vi "ConfigParseProgram.vi"(8 "error in (no error)":errorcluster, 10 "node result array":refnum<k20>[](array[refnum])) -> (0 "error out":errorcluster, 3 "Program Array":string[][](array[string]))   [LabVIEW 2018, in "Config.lvlib"]
uses:
  Config.lvlib
  <vilib>/xml/NI_XML.lvlib
  <resource>/objmgr/DOMUserDefRef.rc
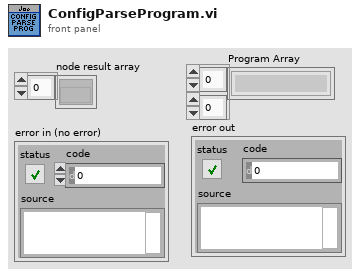
[diagram p1: front panel]
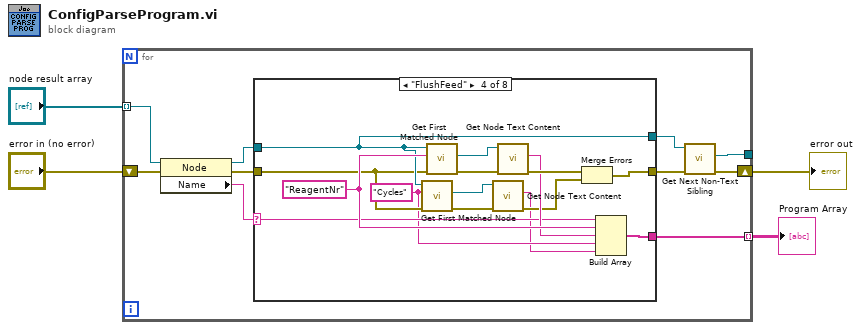
[diagram p0: block diagram]
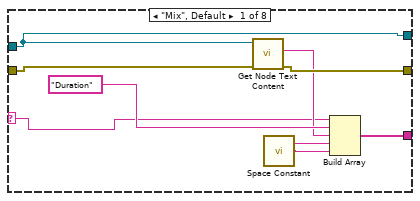
[diagram p2: hidden frame]
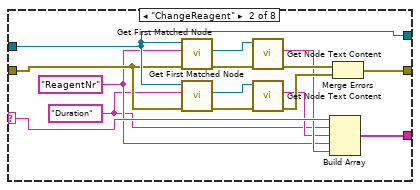
[diagram p3: hidden frame]
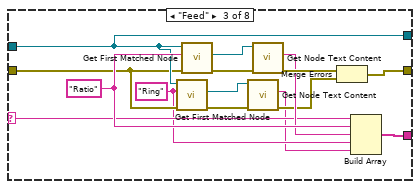
[diagram p4: hidden frame]
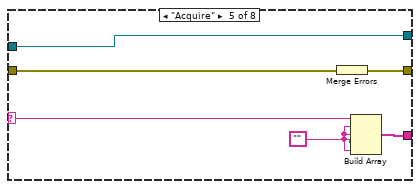
[diagram p5: hidden frame]
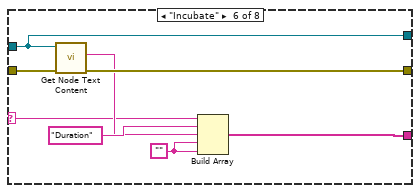
[diagram p6: hidden frame]
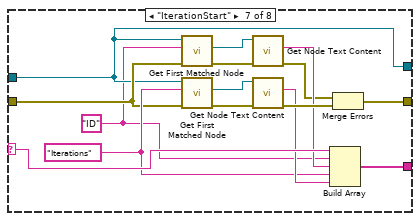
[diagram p7: hidden frame]
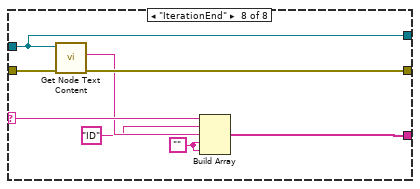
[diagram p8: hidden frame]
diagram:
  n1 = for {
    shift-right: [w5] -> w1
    shift-left: "error in (no error)" -> [w10]
    tunnel: [w6] -> w2 mode=indexing
    tunnel: "node result array" -> [w14] mode=indexing
    tunnel: [w7] -> _
    n2 = property class="Node"(reference=w14, error in=w10) -> (reference out=w11:refnum<k20>, error out=w12:errorcluster, "Name"=w13:string)
    n3 = case shown="\"FlushFeed\"" w13 {
      selector: w13 -> [w17 w28 w46 w61 w71 w78 w92 w102]
      tunnel: w12 -> [w21 w36 w41 w56 w69 w75 w86 w100]
      tunnel: w11 -> [w22 w37 w42 w57 w73 w76 w85 w101]
      tunnel: [w22 w37 w42 w57 w73 w76 w85 w101] -> w9
      tunnel: [w20 w29 w49 w64 w72 w81 w93 w99] -> w8
      tunnel: [w16 w27 w45 w60 w70 w77 w91 w104] -> w6
      frame "Mix", Default {
        n4 = call <vilib>:"Get Node Text Content.vi"("error in (no error)"=w21, "node in"=w22) -> ("error out"=w20:errorcluster, "node text"=w18:string)  [unwired: 7 in, 1 out]
        n5 = call <vilib>:"Space Constant.vi"() -> ("String"=w15:string)
        n6 = Build Array(w17, "Duration" ("XPath expression"), w18, w15, w15) -> (w16:string[])
      }
      frame "ChangeReagent" {
        w23 = "Duration" ("XPath expression")
        w25 = "ReagentNr" ("XPath expression")
        n7 = call <vilib>:"Get First Matched Node.vi"("error in (no error)"=w36, "XPath expression"=w25, "node in"=w37) -> ("error out"=w35:errorcluster, "node result"=w34:refnum<k20>)  [unwired: 6 in, 1 out]
        n8 = call <vilib>:"Get First Matched Node.vi"("error in (no error)"=w36, "XPath expression"=w23, "node in"=w37) -> ("error out"=w33:errorcluster, "node result"=w32:refnum<k20>)  [unwired: 6 in, 1 out]
        n9 = call <vilib>:"Get Node Text Content.vi"("error in (no error)"=w35, "node in"=w34) -> ("error out"=w31:errorcluster, "node text"=w26:string)  [unwired: 7 in, 1 out]
        n10 = call <vilib>:"Get Node Text Content.vi"("error in (no error)"=w33, "node in"=w32) -> ("error out"=w30:errorcluster, "node text"=w24:string)  [unwired: 7 in, 1 out]
        n11 = Build Array(w28, w23, w24, w25, w26) -> (w27:string[])
        n12 = Merge Errors(w31, w30) -> (w29:errorcluster)
      }
      frame "Feed" {
        w39 = "Ring" ("XPath expression")
        w48 = "Ratio" ("XPath expression")
        n13 = call <vilib>:"Get First Matched Node.vi"("error in (no error)"=w41, "XPath expression"=w39, "node in"=w42) -> ("error out"=w44:errorcluster, "node result"=w43:refnum<k20>)  [unwired: 6 in, 1 out]
        n14 = call <vilib>:"Get First Matched Node.vi"("error in (no error)"=w41, "XPath expression"=w48, "node in"=w42) -> ("error out"=w52:errorcluster, "node result"=w51:refnum<k20>)  [unwired: 6 in, 1 out]
        n15 = call <vilib>:"Get Node Text Content.vi"("error in (no error)"=w44, "node in"=w43) -> ("error out"=w40:errorcluster, "node text"=w38:string)  [unwired: 7 in, 1 out]
        n16 = call <vilib>:"Get Node Text Content.vi"("error in (no error)"=w52, "node in"=w51) -> ("error out"=w50:errorcluster, "node text"=w47:string)  [unwired: 7 in, 1 out]
        n17 = Merge Errors(w50, w40) -> (w49:errorcluster)
        n18 = Build Array(w46, w48, w47, w39, w38) -> (w45:string[])
      }
      frame "FlushFeed" {
        w54 = "Cycles" ("XPath expression")
        w63 = "ReagentNr" ("XPath expression")
        n19 = call <vilib>:"Get First Matched Node.vi"("error in (no error)"=w56, "XPath expression"=w54, "node in"=w57) -> ("error out"=w59:errorcluster, "node result"=w58:refnum<k20>)  [unwired: 6 in, 1 out]
        n20 = call <vilib>:"Get First Matched Node.vi"("error in (no error)"=w56, "XPath expression"=w63, "node in"=w57) -> ("error out"=w67:errorcluster, "node result"=w66:refnum<k20>)  [unwired: 6 in, 1 out]
        n21 = call <vilib>:"Get Node Text Content.vi"("error in (no error)"=w59, "node in"=w58) -> ("error out"=w55:errorcluster, "node text"=w53:string)  [unwired: 7 in, 1 out]
        n22 = call <vilib>:"Get Node Text Content.vi"("error in (no error)"=w67, "node in"=w66) -> ("error out"=w65:errorcluster, "node text"=w62:string)  [unwired: 7 in, 1 out]
        n23 = Merge Errors(w65, w55) -> (w64:errorcluster)
        n24 = Build Array(w61, w63, w62, w54, w53) -> (w60:string[])
      }
      frame "Acquire" {
        w68 = ""
        n25 = Merge Errors(w69) -> (w72:errorcluster)
        n26 = Build Array(w71, w68, w68, w68, w68) -> (w70:string[])
      }
      frame "Incubate" {
        w74 = "" ("element")
        n27 = call <vilib>:"Get Node Text Content.vi"("error in (no error)"=w75, "node in"=w76) -> ("error out"=w81:errorcluster, "node text"=w79:string)  [unwired: 7 in, 1 out]
        n28 = Build Array(w78, "Duration" ("XPath expression"), w79, w74, w74) -> (w77:string[])
      }
      frame "IterationStart" {
        w83 = "ID" ("XPath expression")
        w89 = "Iterations" ("XPath expression")
        n29 = call <vilib>:"Get First Matched Node.vi"("error in (no error)"=w86, "XPath expression"=w83, "node in"=w85) -> ("error out"=w88:errorcluster, "node result"=w87:refnum<k20>)  [unwired: 6 in, 1 out]
        n30 = call <vilib>:"Get First Matched Node.vi"("error in (no error)"=w86, "XPath expression"=w89, "node in"=w85) -> ("error out"=w96:errorcluster, "node result"=w95:refnum<k20>)  [unwired: 6 in, 1 out]
        n31 = call <vilib>:"Get Node Text Content.vi"("error in (no error)"=w88, "node in"=w87) -> ("error out"=w82:errorcluster, "node text"=w84:string)  [unwired: 7 in, 1 out]
        n32 = call <vilib>:"Get Node Text Content.vi"("error in (no error)"=w96, "node in"=w95) -> ("error out"=w94:errorcluster, "node text"=w90:string)  [unwired: 7 in, 1 out]
        n33 = Build Array(w92, w83, w84, w89, w90) -> (w91:string[])
        n34 = Merge Errors(w82, w94) -> (w93:errorcluster)
      }
      frame "IterationEnd" {
        w103 = ""
        n35 = call <vilib>:"Get Node Text Content.vi"("error in (no error)"=w100, "node in"=w101) -> ("error out"=w99:errorcluster, "node text"=w98:string)  [unwired: 7 in, 1 out]
        n36 = Build Array(w102, "ID", w98, w103, w103) -> (w104:string[])
      }
    }
    n37 = call <vilib>:"Get Next Non-Text Sibling.vi"("error in (no error)"=w8, "node in"=w9) -> ("error out"=w5:errorcluster, "sibling node"=w7:refnum<k20>)  [unwired: 6 in, 2 out]
  }
  "Program Array" <- w2
  "error out" <- w1
